vi "storage.reader.vi"(7 "Data Source RID":string, 8 "error in":errorcluster, 9 "Points":T1(array[cluster]), 10 "Channel":string, 11 "Nominal Client in":refnum<class "Nominal Client.lvclass">) -> (0 "error out":errorcluster, 2 "Response body":string, 3 "Nominal Client out":refnum<class "Nominal Client.lvclass">, 4 "Response Headers":refnum<class "Response Headers.lvclass">)   [LabVIEW 2020, in "Nominal Client.lvclass"]
uses:
  Nominal Client.lvclass
  <vilib>/addons/_JKI.lib/REST Client/classes/Response Headers/Response Headers.lvclass
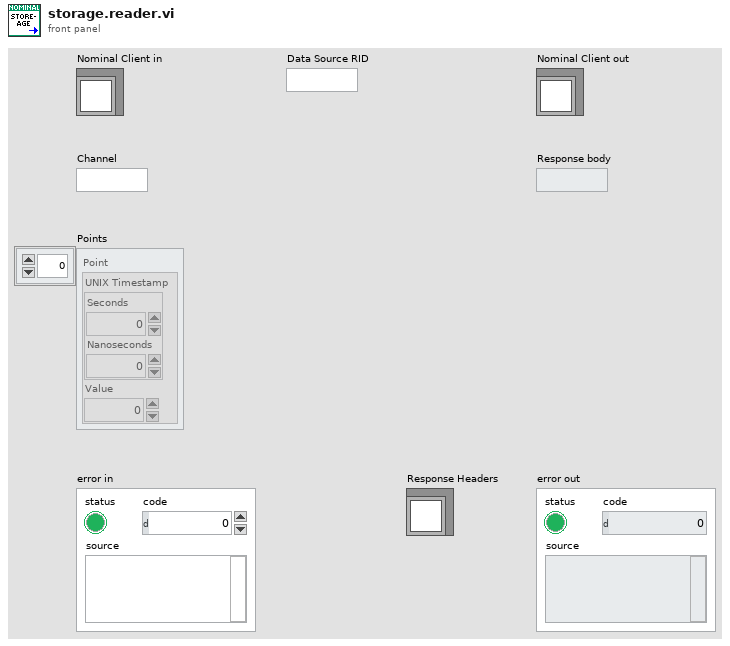
[diagram p1: front panel]
types:
  T1 = cluster{"UNIX Timestamp":cluster{"Seconds":i64, "Nanoseconds":i64}, "Value":dbl}[]
  T2 = cluster{"batches":cluster{"channel":string, "points":cluster{"type":string, "double":cluster{"timestamp":cluster{"seconds":i32, "nanos":i32}, "value":dbl}[]}}[], "dataSourceRid":string}
  T3 = cluster{cluster{"Channel":string, cluster{"type":string, "Points":cluster{"UNIX Timestamp":cluster{"Seconds":i64, "Nanoseconds":i64}, "Value":dbl}[]}}[], "Data Source RID":string}
  T4 = cluster{"batches":cluster{"channel":string, "points":cluster{"type":string, "double":cluster{"timestamp":cluster{"nanos":i32, "seconds":i32}, "value":dbl}[]}}[], "dataSourceRid":string}
  T5 = cluster{"type":string, "Points":cluster{"UNIX Timestamp":cluster{"Seconds":i64, "Nanoseconds":i64}, "Value":dbl}[]}
  T6 = cluster{"Channel":string, cluster{"type":string, "Points":cluster{"UNIX Timestamp":cluster{"Seconds":i64, "Nanoseconds":i64}, "Value":dbl}[]}}
  T7 = cluster{"Channel":string, cluster{"type":string, "Points":cluster{"UNIX Timestamp":cluster{"Seconds":i64, "Nanoseconds":i64}, "Value":dbl}[]}}[]
  T8 = cluster{"batches":cluster{"channel":string, "points":cluster{"type":string, "double":cluster{"timestamp":cluster{"nanos":i32, "seconds":i32}, "value":string}[]}}[], "dataSourceRid":string}
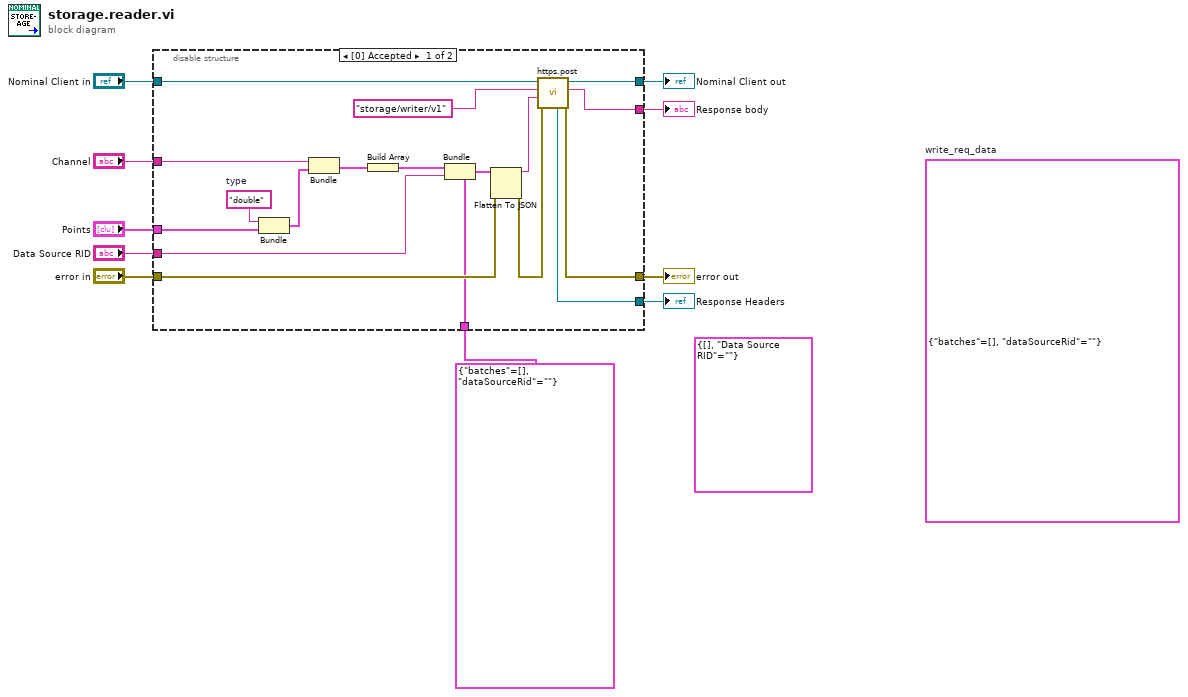
[diagram p0: block diagram]
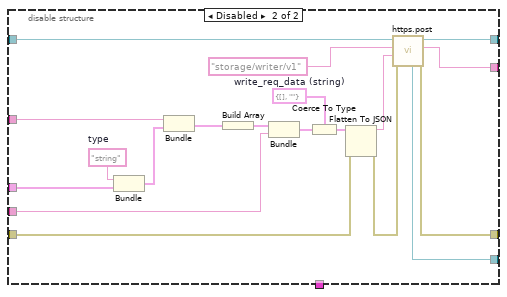
[diagram p2: hidden frame]
diagram:
  (unwired) T3 {[], "Data Source RID"=""} ("output cluster")
  (unwired) T4 {"batches"=[], "dataSourceRid"=""}  # write_req_data
  n1 = disable-structure shown="[0] Accepted" {
    disable-tunnel: "Nominal Client in" -> [w28 w47]
    disable-tunnel: [w27 w46] -> w9
    disable-tunnel: [w25 w44] -> w8
    disable-tunnel: [w24 w43] -> w7
    disable-tunnel: [w23 w42] -> w6
    disable-tunnel: "Points" -> [w13 w29]
    disable-tunnel: "Channel" -> [w20 w39]
    disable-tunnel: "Data Source RID" -> [w17 w36]
    disable-tunnel: "error in" -> [w16 w32]
    disable-tunnel: T2 {"batches"=[], "dataSourceRid"=""} ("output cluster") -> [w11 _]
    frame Enabled {
      w22 = "double"  # type
      n2 = Bundle("type"=w22, "Points"=w13) -> (w21:T5)  [unwired: 1 in]
      n3 = Bundle("Channel"=w20, w21) -> (w19:T6)  [unwired: 1 in]
      n4 = Build Array(w19) -> (w18:T7)
      n5 = Bundle(cluster=w11, "batches"=w18, "dataSourceRid"=w17) -> (w12:T2)
      n6 = Flatten To JSON(anything=w12, error in (no error)=w16) -> (JSON string=w14:string, 11:w15:errorcluster)  [unwired: 1 in]
      n7 = call "https.post.vi"("error in"=w15, "Request body"=w14, "Path"="storage/writer/v1", "Nominal Client in"=w28) -> ("error out"=w25:errorcluster, "Response"=w23:string, "Nominal Client out"=w27:refnum<class "Nominal Client.lvclass">, "Response Headers"=w24:refnum<class "Response Headers.lvclass">)  [unwired: 4 in]
    }
    frame Disabled {
      w34 = T8 {"batches"=[], "dataSourceRid"=""}  # write_req_data (string)
      w41 = "string"  # type
      n8 = Bundle("type"=w41, "Points"=w29) -> (w40:T5)  [unwired: 1 in]
      n9 = Bundle("Channel"=w39, w40) -> (w38:T6)  [unwired: 1 in]
      n10 = Build Array(w38) -> (w37:T7)
      n11 = Bundle(w37, "Data Source RID"=w36) -> (w35:T3)  [unwired: 1 in]
      n12 = Coerce To Type(0:w35, 1:w34) -> (2:w33:T8)
      n13 = Flatten To JSON(anything=w33, error in (no error)=w32) -> (JSON string=w30:string, 11:w31:errorcluster)  [unwired: 1 in]
      n14 = call "https.post.vi"("error in"=w31, "Request body"=w30, "Path"="storage/writer/v1", "Nominal Client in"=w47) -> ("error out"=w44:errorcluster, "Response"=w42:string, "Nominal Client out"=w46:refnum<class "Nominal Client.lvclass">, "Response Headers"=w43:refnum<class "Response Headers.lvclass">)  [unwired: 4 in]
    }
  }
  "Nominal Client out" <- w9
  "error out" <- w8
  "Response body" <- w6
  "Response Headers" <- w7
